vi "Logging.vi"(8 "error in (no error)":errorcluster, 11 "Node Ptr":T1 format="%.0x") -> (0 "error out":errorcluster)   [LabVIEW 2020, in "AIM ARINC 664 System Explorer.lvlib" / "Implementation.lvlib"]
uses:
  Implementation.lvlib
  <vilib>/NI VeriStand/Custom Device API/Custom Device Item Ref.ctl
  Shared/loggingThreshold_types.ctl
  <vilib>/NI VeriStand/Custom Device API/Custom Device API.lvlib
  Scripting/AIM ARINC 664 Scripting.lvlib
panel:
  in  "Enable Logging":bool
  in  "Segment Files By":u16(ring) items=["Time", "Size"]
  in  "Free drive percent":dbl=10.0 caption="percent(%)"
  in  "Segment Files":bool caption="Segment into Multiple Files"
  in  "threshold":dbl=10.0 caption="Create new file when the time duration exceeds [sec]"
  in  "Stop on HDD space":bool caption="Stop Logging when hard drive free space is less than"
  in  "Timestamp Filename":bool
  in  "File Name":string
  out "Example Log File Path":string
  in  "Log Directory":string
  in  "SHDocVw.IWebBrowser":refnum<k7>(container)
  in  "General Header":cluster{"Section Name":string}={"Section Name"="General Custom Device Settings"}
  in  "Description":string
  in  "Name":string
  # ".pcap"
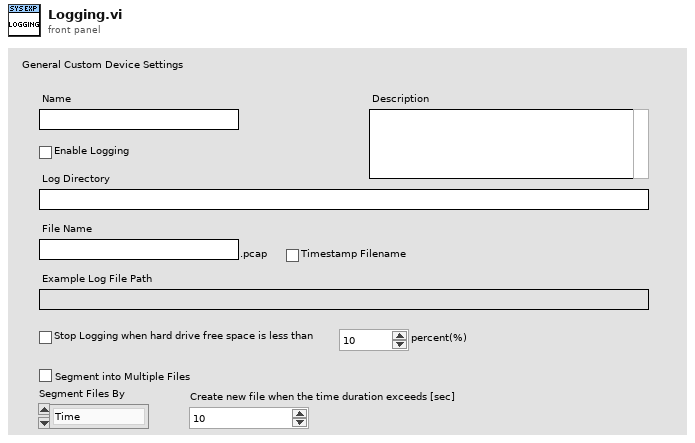
[diagram p1: front panel]
types:
  T1 = typedef "Custom Device API.lvlib/Custom Device Item Ref.ctl" = u64
  T2 = typedef "loggingThreshold_types.ctl" = cluster{"Segmentation Threshold":dbl, "Disk Space Percentage":dbl, "Check Disk Space":bool, "Segment File":bool, "Segment Files By":u16}
  T3 = typedef "logFileInfo_types.ctl" = cluster{"Log Directory":string, "Base Name":string, "Timestamp":bool, "Enabled":bool}
  T4 = typedef "Custom Device API.lvlib/Custom Device Target Type.ctl" = enum16{"PharLap", "VxWorks", "Windows", "Linux_32_ARM", "Linux_x64"}
  T5 = typedef "Custom Device API.lvlib/Custom Device Item Info.ctl" = cluster{"Name":string, "Is Channel":bool, "GUID":string, "Is Waveform":bool}
  T6 = typedef "Custom Device API.lvlib/Custom Device Commands.ctl" = enum16{"Default", "Item renamed", "Shutdown", "Dynamic button pressed"}
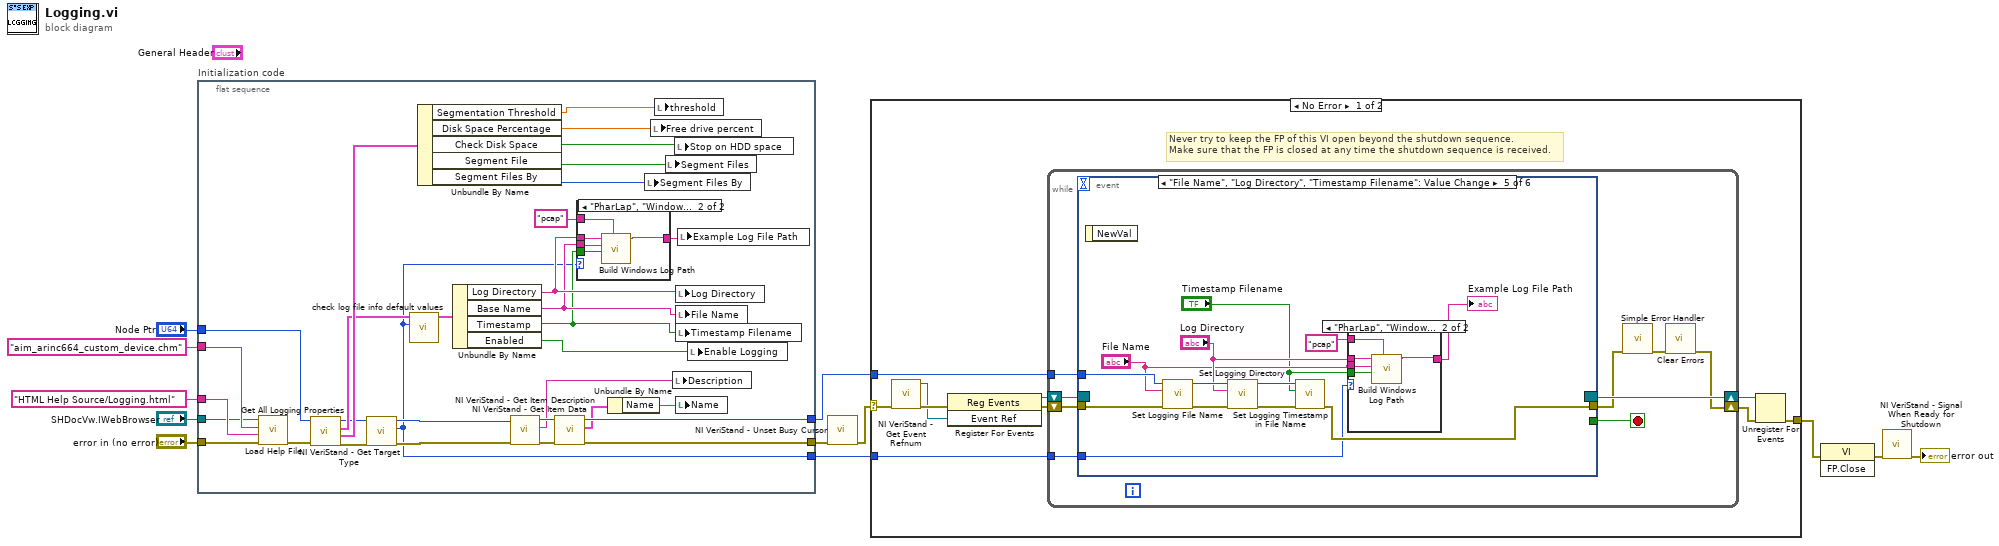
[diagram p0: block diagram]
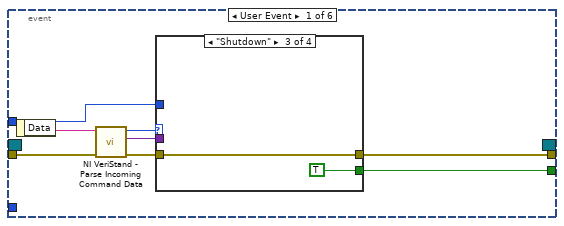
[diagram p2: hidden frame]
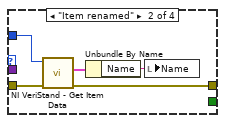
[diagram p4: hidden frame]
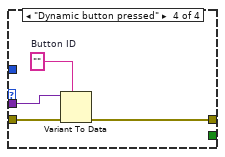
[diagram p5: hidden frame]
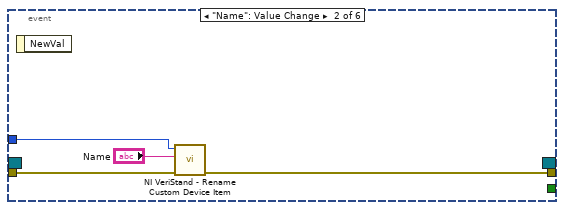
[diagram p6: hidden frame]
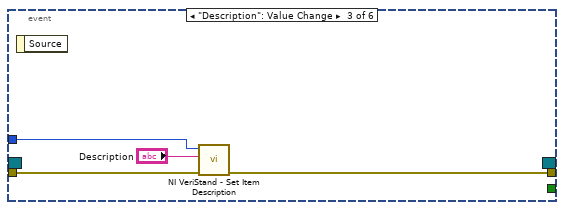
[diagram p7: hidden frame]
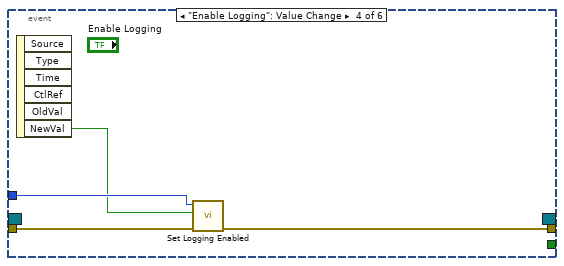
[diagram p8: hidden frame]
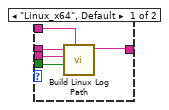
[diagram p9: hidden frame]
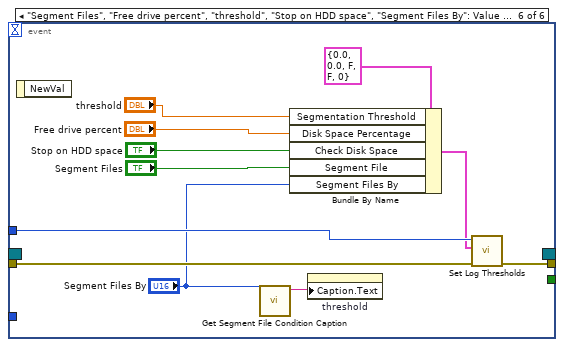
[diagram p10: hidden frame]
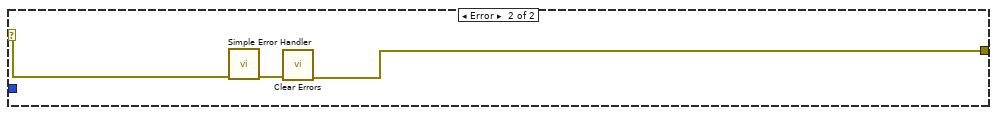
[diagram p11: hidden frame]
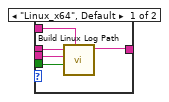
[diagram p12: hidden frame]
diagram:
  n1 = flat-sequence "Initialization code" {
    tunnel: "error in (no error)" -> [w37]
    tunnel: "Node Ptr" -> [w32]
    tunnel: [w40] -> w8
    tunnel: [w44] -> w5
    tunnel: "SHDocVw.IWebBrowser" -> [w34]
    tunnel: "HTML Help Source/Logging.html" ("HTML File") -> [w35]
    tunnel: "aim_arinc664_custom_device.chm" ("CD_CHM_FileName") -> [w36]
    tunnel: [w13] -> w1
    frame #0 {
      n2 = call "Load Help File.vi"("error in (no error)"=w37, "HTML File to Load"=w35, "Main CHM File"=w36, "Browser"=w34) -> ("error out"=w31:errorcluster)  [unwired: 6 in, 1 out]
      n3 = call "Get All Logging Properties.vi"("error in"=w31, "logging ref"=w32) -> ("error out"=w16:errorcluster, "log thresholds"=w30:T2, "log file info"=w20:T3, "logging ref out"=w17:T1)  [unwired: 6 in]
      n4 = call <vilib>:"NI VeriStand - Get Target Type.vi"("error in (no error)"=w16, "Item Ref in"=w17) -> ("error out"=w15:errorcluster, "Target Type"=w13:T4, "Item Ref out"=w14:T1)  [unwired: 7 in]
      n5 = call "check log file info default values.vi"("Target Type"=w13, "log file info in"=w20) -> ("log file info out"=w19:T3)  [unwired: 9 in]
      n6 = Unbundle By Name(w30) -> ("Segmentation Threshold"=w22:dbl, "Disk Space Percentage"=w24:dbl, "Check Disk Space"=w25:bool, "Segment File"=w26:bool, "Segment Files By"=w23:u16)
      n7 = Unbundle By Name(w19) -> ("Log Directory"=w29:string, "Base Name"=w28:string, "Timestamp"=w27:bool, "Enabled"=w18:bool)
      n8 = call <vilib>:"NI VeriStand - Get Item Description.vi"("error in (no error)"=w15, "Item Ref in"=w14) -> ("error out"=w42:errorcluster, "Description"=w38:string, "Item Ref out"=w43:T1)  [unwired: 7 out]
      n9 = call <vilib>:"NI VeriStand - Get Item Data.vi"("error in (no error)"=w42, "Item Ref in"=w43) -> ("error out"=w40:errorcluster, "Item Info"=w41:T5, "Item Ref out"=w44:T1)  [unwired: 7 out]
      n10 = case shown="\"PharLap\", \"Windows\"" w13 {
        tunnel: [w45 w54] -> w33
        tunnel: w29 -> [w48 w52]
        tunnel: w28 -> [w47 w51]
        tunnel: w27 -> [w46 w50]
        tunnel: "pcap" ("Extension") -> [w49 w53]
        frame "Linux_x64", Default {
          n11 = call "Build Linux Log Path.vi"("Extension"=w49, "Timestamp"=w46, "Name"=w47, "Log File Directory"=w48) -> ("Log File Path"=w45:string)  [unwired: 6 in, 1 out]
        }
        frame "PharLap", "Windows" {
          n12 = call "Build Windows Log Path.vi"("Extension"=w53, "Timestamp"=w50, "Name"=w51, "Log File Directory"=w52) -> ("Log File Path"=w54:string)  [unwired: 6 in, 1 out]
        }
      }
      n13 = Unbundle By Name(w41) -> ("Name"=w39:string)
      n14 = local write "Segment Files By"(w23) -> ()
      n15 = local write "Free drive percent"(w24) -> ()
      n16 = local write "threshold"(w22) -> ()
      n17 = local write "Segment Files"(w26) -> ()
      n18 = local write "Description"(w38) -> ()
      n19 = local write "Stop on HDD space"(w25) -> ()
      n20 = local write "Log Directory"(w29) -> ()
      n21 = local write "File Name"(w28) -> ()
      n22 = local write "Timestamp Filename"(w27) -> ()
      n23 = local write "Name"(w39) -> ()
      n24 = local write "Example Log File Path"(w33) -> ()
      n25 = local write "Enable Logging"(w18) -> ()
    }
  }
  n26 = call <vilib>:"NI VeriStand - Unset Busy Cursor.vi"("error in (no error)"=w8) -> ("error out"=w7:errorcluster)  [unwired: 10 out]
  n27 = case shown="No Error" w7 {
    selector: w7 -> [w56 w142]
    tunnel: [w61 w140] -> w12
    tunnel: w5 -> [w57 _]
    tunnel: w1 -> [w55 _]
    frame No Error {
      # "Never try to keep the FP of this VI open beyond the shutdown sequence.\nMake sure that the FP is closed at any time the shutdown sequence is received."
      n28 = call <vilib>:"NI VeriStand - Get Event Refnum.vi"("error in (no error)"=w56) -> ("error out"=w64:errorcluster, "Event Ref"=w60:refnum<user-event>)  [unwired: 9 out]
      n29 = register-events(error in=w64, w60) -> (reference out=w58:refnum<event-registration>, error out=w59:errorcluster)  [unwired: 1 in]
      n30 = while {
        tunnel: w57 -> [w69]
        shift-right: [w66] -> w62
        shift-left: w59 -> [w72]
        shift-right: [w73] -> w63
        shift-left: w58 -> [w71]
        tunnel: w55 -> [w65]
        stop <- w70 stop-if-true
        n31 = event shown="[4] \"File Name\", \"Log Directory\", \"Timestamp Filename\": Value Change" {
          selector: w71 -> [_ _ _ _ _ _]
          dyn-events: [_ _ _ _ _ _] -> w73
          timeout: _ -> [_ _ _ _ _ _]
          tunnel: w72 -> [w81 w97 w100 w105 w118 w139]
          tunnel: [w77 _ _ _ _ _] -> w70
          tunnel: [w76 w96 w99 w104 w112 w137] -> w68
          tunnel: w69 -> [w75 w95 w101 w103 w117 w138]
          tunnel: w65 -> [_ _ _ _ w111 _]
          event User Event {
            n32 = event-data() -> ("Data"=w80:string)  [unwired: 1 out]
            n33 = call <vilib>:"NI VeriStand - Parse Incoming Command Data.vi"("error in (no error)"=w81, "Incoming data"=w80) -> ("error out"=w79:errorcluster, "Outgoing data"=w74:variant, "Action"=w78:T6)  [unwired: 7 out]
            n34 = case shown="\"Shutdown\"" w78 {
              tunnel: w79 -> [w82 w87 w88 w93]
              tunnel: [_ _ TRUE _] -> w77
              tunnel: [w82 w84 w88 w90] -> w76
              tunnel: w75 -> [_ w86 _ _]
              tunnel: w74 -> [_ _ _ w92]
              frame "Default", Default {
              }
              frame "Item renamed" {
                n35 = call <vilib>:"NI VeriStand - Get Item Data.vi"("error in (no error)"=w87, "Item Ref in"=w86) -> ("error out"=w84:errorcluster, "Item Info"=w85:T5)  [unwired: 8 out]
                n36 = Unbundle By Name(w85) -> ("Name"=w83:string)
                n37 = local write "Name"(w83) -> ()
              }
              frame "Shutdown" {
              }
              frame "Dynamic button pressed" {
                w91 = ""  # Button ID
                n38 = Variant To Data(error in=w93, type=w91, Variant=w92) -> (error out=w90:errorcluster)  [unwired: 1 out]
              }
            }
          }
          event "Name": Value Change {
            n39 = event-data() -> ()  [unwired: 2 out]
            n40 = call <vilib>:"NI VeriStand - Rename Custom Device Item.vi"("error in (no error)"=w97, "New Name"="Name", "Item Ref in"=w95) -> ("error out"=w96:errorcluster)  [unwired: 1 in, 7 out]
          }
          event "Description": Value Change {
            n41 = event-data() -> ()  [unwired: 2 out]
            n42 = call <vilib>:"NI VeriStand - Set Item Description.vi"("error in (no error)"=w100, "Description"="Description", "Item Ref in"=w101) -> ("error out"=w99:errorcluster)  [unwired: 8 out]
          }
          event "Enable Logging": Value Change {
            n43 = event-data() -> ("NewVal"=w102:bool)  [unwired: 6 out]
            n44 = call "Set Logging Enabled.vi"("error in"=w105, "Value"=w102, "logging ref"=w103) -> ("error out"=w104:errorcluster)  [unwired: 7 in, 1 out]
          }
          event "File Name", "Log Directory", "Timestamp Filename": Value Change {
            n45 = event-data() -> ()  [unwired: 2 out]
            n46 = call "Set Logging File Name.vi"("error in"=w118, "file name"="File Name", "logging ref"=w117) -> ("error out"=w116:errorcluster, "logging ref out"=w115:T1)  [unwired: 7 in]
            n47 = call "Set Logging Directory.vi"("error in"=w116, "Default Value"="Log Directory", "logging ref"=w115) -> ("error out"=w113:errorcluster, "logging ref out"=w114:T1)  [unwired: 7 in]
            n48 = call "Set Logging Timestamp in File Name.vi"("error in"=w113, "Default Value"="Timestamp Filename", "logging ref"=w114) -> ("error out"=w112:errorcluster)  [unwired: 7 in, 1 out]
            n49 = case shown="\"PharLap\", \"Windows\"" w111 {
              tunnel: [w119 w128] -> w108
              tunnel: "Log Directory" -> [w122 w126]
              tunnel: "File Name" -> [w121 w125]
              tunnel: "Timestamp Filename" -> [w120 w124]
              tunnel: "pcap" ("Extension") -> [w123 w127]
              frame "Linux_x64", Default {
                n50 = call "Build Linux Log Path.vi"("Extension"=w123, "Timestamp"=w120, "Name"=w121, "Log File Directory"=w122) -> ("Log File Path"=w119:string)  [unwired: 6 in, 1 out]
              }
              frame "PharLap", "Windows" {
                n51 = call "Build Windows Log Path.vi"("Extension"=w127, "Timestamp"=w124, "Name"=w125, "Log File Directory"=w126) -> ("Log File Path"=w128:string)  [unwired: 6 in, 1 out]
              }
            }
            "Example Log File Path" <- w108
          }
          event "Segment Files", "Free drive percent", "threshold", "Stop on HDD space", "Segment Files By": Value Change {
            n52 = event-data() -> ()  [unwired: 2 out]
            n53 = call "Get Segment File Condition Caption.vi"("Segment Files By"="Segment Files By") -> ("Segment File Size Caption"=w136:string)  [unwired: 10 in]
            n54 = Bundle By Name(cluster=T2 {"Segmentation Threshold"=0.0, "Disk Space Percentage"=0.0, "Check Disk Space"=FALSE, "Segment File"=FALSE, "Segment Files By"=0} ("log thresholds"), "Segmentation Threshold"="threshold", "Disk Space Percentage"="Free drive percent", "Check Disk Space"="Stop on HDD space", "Segment File"="Segment Files", "Segment Files By"="Segment Files By") -> (w131:T2)
            n55 = property on="threshold" class="DigNum (strict)"("Caption.Text"=w136) -> ()  [unwired: 2 in, 2 out]
            n56 = call "Set Log Thresholds.vi"("error in"=w139, "log thresholds"=w131, "logging ref"=w138) -> ("error out"=w137:errorcluster)  [unwired: 7 in, 1 out]
          }
        }
        n57 = call <vilib>:"Simple Error Handler.vi"("error in (no error)"=w68) -> ("error out"=w67:errorcluster)  [unwired: 1 in, 7 out]
        n58 = call <vilib>:"Clear Errors.vi"("error in (no error)"=w67) -> ("error out"=w66:errorcluster)  [unwired: 1 in, 5 out]
      }
      n59 = Unregister For Events(event registration refnum=w63, error in=w62) -> (error out=w61:errorcluster)
    }
    frame Error {
      n60 = call <vilib>:"Simple Error Handler.vi"("error in (no error)"=w142) -> ("error out"=w141:errorcluster)  [unwired: 1 in, 7 out]
      n61 = call <vilib>:"Clear Errors.vi"("error in (no error)"=w141) -> ("error out"=w140:errorcluster)  [unwired: 1 in, 5 out]
    }
  }
  n62 = invoke class="VI" method="FP.Close"(error in=w12) -> (error out=w11:errorcluster)  [unwired: 2 in, 2 out]
  n63 = call <vilib>:"NI VeriStand - Signal When Ready for Shutdown.vi"("error in (no error)"=w11) -> ("error out"=→"error out":errorcluster)  [unwired: 10 out]
